vi "Export New Records.vi"(8 "error IN":errorcluster, 11 "Site":string) -> (0 "error out":errorcluster)   [LabVIEW 2015]
uses:
  <vilib>/addons/database/Connection.llb/DB Tools Open Connec (Path).vi
  <vilib>/addons/database/Connection.llb/Conn Execute.vi
  <vilib>/addons/database/Recordset.llb/Rec Destroy - Connection.vi
  <vilib>/addons/database/NI_Database_API.lvlib
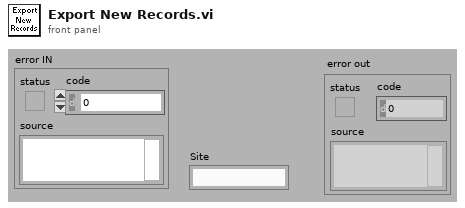
[diagram p1: front panel]
types:
  T1 = typedef "NI_Database_API.lvlib/Conn ObjectReference.ctl" = refnum<k1>
  T2 = typedef "NI_Database_API.lvlib/Rec ObjectReference.ctl" = refnum<k1>
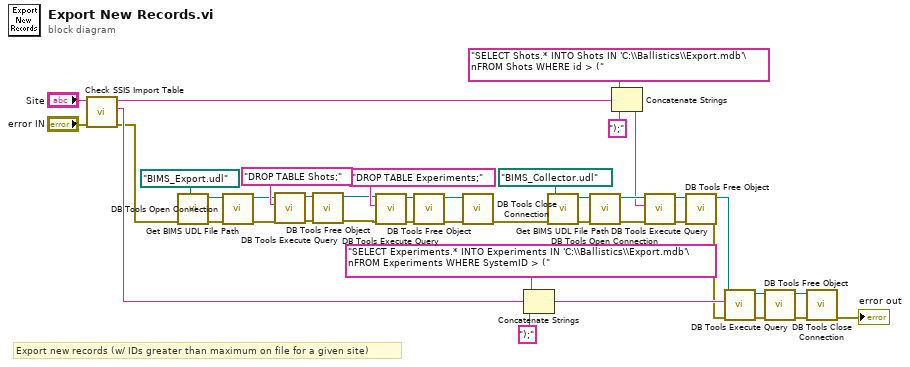
[diagram p0: block diagram]
diagram:
  # "Export new records (w/ IDs greater than maximum on file for a given site)"
  n1 = call "Check SSIS Import Table.vi"("error IN"="error IN", "Site"="Site") -> ("error OUT"=w5:errorcluster, "max expt rec"=w25:string, "max shot id rec"=w9:string)  [unwired: 7 out]
  n2 = call "Get BIMS UDL File Path.vi"("error in"=w5, "UDL file name"=path "BIMS_Export.udl") -> ("error out"=w4:errorcluster, "Full UDL file path"=w37:path)  [unwired: 4 out]
  n3 = call-poly <vilib>:"DB Tools Open Connection.vi"("error in (no error)"=w4, "connection information"=w37) -> ("error out"=w21:errorcluster, "connection reference"=w20:T1)  [unwired: 3 in, 3 out]
  n4 = call-poly <vilib>:"DB Tools Execute Query.vi"("error in (no error)"=w21, "SQL query"="DROP TABLE Shots;", "connection reference"=w20) -> ("error out"=w16:errorcluster, "recordset reference"=w22:T2)  [unwired: 2 in, 3 out]
  n5 = call-poly <vilib>:"DB Tools Free Object.vi"("error in (no error)"=w16, "recordset reference"=w22) -> ("error out"=w18:errorcluster, "connection reference"=w19:T1)  [unwired: 8 out]
  n6 = call-poly <vilib>:"DB Tools Execute Query.vi"("error in (no error)"=w18, "SQL query"="DROP TABLE Experiments;", "connection reference"=w19) -> ("error out"=w39:errorcluster, "recordset reference"=w36:T2)  [unwired: 2 in, 3 out]
  n7 = call-poly <vilib>:"DB Tools Free Object.vi"("error in (no error)"=w39, "recordset reference"=w36) -> ("error out"=w29:errorcluster, "connection reference"=w24:T1)  [unwired: 8 out]
  n8 = call <vilib>:"DB Tools Close Connection.vi"("error in (no error)"=w29, "connection reference"=w24) -> ("error out"=w7:errorcluster)  [unwired: 5 out]
  n9 = Concatenate Strings("SELECT Experiments.* INTO Experiments IN 'C:\\Ballistics\\Export.mdb'\nFROM Experiments WHERE SystemID > (" ("string"), w25, ");" ("message")) -> (w27:string)
  n10 = call "Get BIMS UDL File Path.vi"("error in"=w7, "UDL file name"=path "BIMS_Collector.udl") -> ("error out"=w6:errorcluster, "Full UDL file path"=w40:path)  [unwired: 4 out]
  n11 = call-poly <vilib>:"DB Tools Open Connection.vi"("error in (no error)"=w6, "connection information"=w40) -> ("error out"=w14:errorcluster, "connection reference"=w11:T1)  [unwired: 3 in, 3 out]
  n12 = Concatenate Strings("SELECT Shots.* INTO Shots IN 'C:\\Ballistics\\Export.mdb'\nFROM Shots WHERE id > (" ("string"), w9, ");" ("message")) -> (w10:string)
  n13 = call-poly <vilib>:"DB Tools Execute Query.vi"("error in (no error)"=w14, "SQL query"=w10, "connection reference"=w11) -> ("error out"=w15:errorcluster, "recordset reference"=w8:T2)  [unwired: 2 in, 3 out]
  n14 = call-poly <vilib>:"DB Tools Free Object.vi"("error in (no error)"=w15, "recordset reference"=w8) -> ("error out"=w13:errorcluster, "connection reference"=w12:T1)  [unwired: 8 out]
  n15 = call-poly <vilib>:"DB Tools Execute Query.vi"("error in (no error)"=w13, "SQL query"=w27, "connection reference"=w12) -> ("error out"=w34:errorcluster, "recordset reference"=w35:T2)  [unwired: 2 in, 3 out]
  n16 = call-poly <vilib>:"DB Tools Free Object.vi"("error in (no error)"=w34, "recordset reference"=w35) -> ("error out"=w31:errorcluster, "connection reference"=w32:T1)  [unwired: 8 out]
  n17 = call <vilib>:"DB Tools Close Connection.vi"("error in (no error)"=w31, "connection reference"=w32) -> ("error out"=→"error out":errorcluster)  [unwired: 5 out]
